vi "Loader.vi"(9 "Loader Name":string, 10 "PID":u32) -> ()   [LabVIEW 2021, in "CIFPluginLoader.lvclass"]
uses:
  CIFPluginLoader.lvclass
  CIFUtilities/CIFLogs/Typedef/Message Type.ctl
  gRPC/CIF_PluginLoader_server/RPC Messages/cif_common_Empty.ctl
  gRPC/CIF_PluginLoader_server/RPC Messages/cif_common_Status.ctl
  CIFPluginLoader.lvclass/CIFPluginLoader.ctl
  gRPC/CIF_PluginLoader_server/RPC Messages/cif_manager_LoaderStatus.ctl
  gRPC/CIF_PluginLoader_server/RPC Messages/cif_manager_LoaderInfo.ctl
  gRPC/CIF_PluginLoader_server/RPC Messages/cif_manager_LoaderType.ctl
  <vilib>/gRPC/LabVIEW gRPC Servicer/Servicer/Servicer.lvclass
  CIFUtilities/CIFLogs/CIFLogs.lvlib
  CIFUtilities/CIFConfigurationFile/typedef/Location Type.ctl
  CIFUtilities/CIFConfigurationFile/CIF Configuration File.lvlib
  <vilib>/Utility/LVLibp/NI_PackedLibraryUtility.lvlib
  gRPC/CIF_PluginLoader_server/RPC Service/PluginLoader/PluginLoader.lvclass
  gRPC/CIF_PluginLoader_server/CIF_PluginLoader_server.lvlib
  gRPC/CIF_PluginLoader_server/RPC Messages/cif_common_Version.ctl
  gRPC/CIF_PluginLoader_server/RPC Messages/cif_manager_PluginMetadata.ctl
  gRPC/CIF_PluginLoader_server/RPC Messages/cif_pluginloader_DiscoveredPlugin.ctl
  gRPC/CIF_PluginLoader_server/RPC Messages/cif_pluginloader_DiscoveredPlugins.ctl
  gRPC/CIF_Plugin_Loader_Client_Wrapper/CIFPluginLoaderClientWrapper.lvlib
panel:
  out "error out":errorcluster
  in  "stop":bool
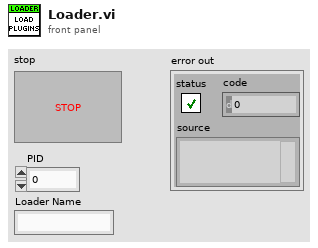
[diagram p1: front panel]
types:
  T1 = typedef "CIFLogs.lvlib/Message Type.ctl" = enum16{"Error", "Information", "Print Terminal", "Configuration"}
  T2 = typedef "CIF_PluginLoader_server.lvlib/cif_pluginloader_DiscoveredPlugins.ctl" = cluster{"discovered_plugins":T3[], "status":T6}
  T3 = typedef "CIF_PluginLoader_server.lvlib/cif_pluginloader_DiscoveredPlugin.ctl" = cluster{"file_path":string, "file_name":string, "plugin_type":string, "plugin_version":T4, "plugin_metadata":T5}
  T4 = typedef "CIF_PluginLoader_server.lvlib/cif_common_Version.ctl" = cluster{"major":u32, "minor":u32, "fix":u32, "build":u32}
  T5 = typedef "CIF_PluginLoader_server.lvlib/cif_manager_PluginMetadata.ctl" = cluster{"description":string, "history":string, "author":string}
  T6 = typedef "CIF_PluginLoader_server.lvlib/cif_common_Status.ctl" = cluster{"code":i32, "message":string}
  T7 = typedef "CIF Configuration File.lvlib/Location Type.ctl" = enum16{"Config File", "Manager", "Protos", "Plugins", "UI Plugins", "Logs", "Orchestrations"}
  T8 = typedef "CIF_PluginLoader_server.lvlib/cif_common_Empty.ctl" = cluster{"void":string}
  T9 = typedef "CIF_PluginLoader_server.lvlib/cif_manager_LoaderStatus.ctl" = cluster{"loader_info":T10, "grpc_port":i32, "pid":u32}
  T10 = typedef "CIF_PluginLoader_server.lvlib/cif_manager_LoaderInfo.ctl" = cluster{"loader_type":T11, "loader_name":string}
  T11 = typedef "CIF_PluginLoader_server.lvlib/cif_manager_LoaderType.ctl" = enum32{"LOADERTYPE_UNKNOWN", "LOADERTYPE_LABVIEW"}
  T12 = typedef "grpc-lvsupport-release.lvlib/grpcId.ctl" = u64
  T13 = typedef "CIF_PluginLoader_server.lvlib/cif_pluginloader_DiscoverCommand.ctl" = cluster{"update_metadata":bool}
  T14 = typedef "trash_Discovered Plugin.ctl" = cluster{"Filename":string, "Plugin Type":string, "Qualified name":string, "Version":T15, "Plugin Metadata":T16}
  T15 = typedef "CIFCoreCommon.lvlib/Version.ctl" = cluster{"Major":i32, "Minor":i32, "Fix":i32, "Build":i32}
  T16 = typedef "trash_Plugin Metadata.ctl" = cluster{"Description":string, "History":string, "Author":string}
  T17 = typedef "CIF_PluginLoader_server.lvlib/cif_pluginloader_LoadConfig.ctl" = cluster{"plugin_name":T18, "path":string}
  T18 = typedef "CIF_PluginLoader_server.lvlib/cif_manager_PluginName.ctl" = cluster{"plugin_name":string}
  T19 = typedef "CIFPluginLoader.lvclass/Loaded Plugin Map.ctl" = map{string, refnum<vi>}
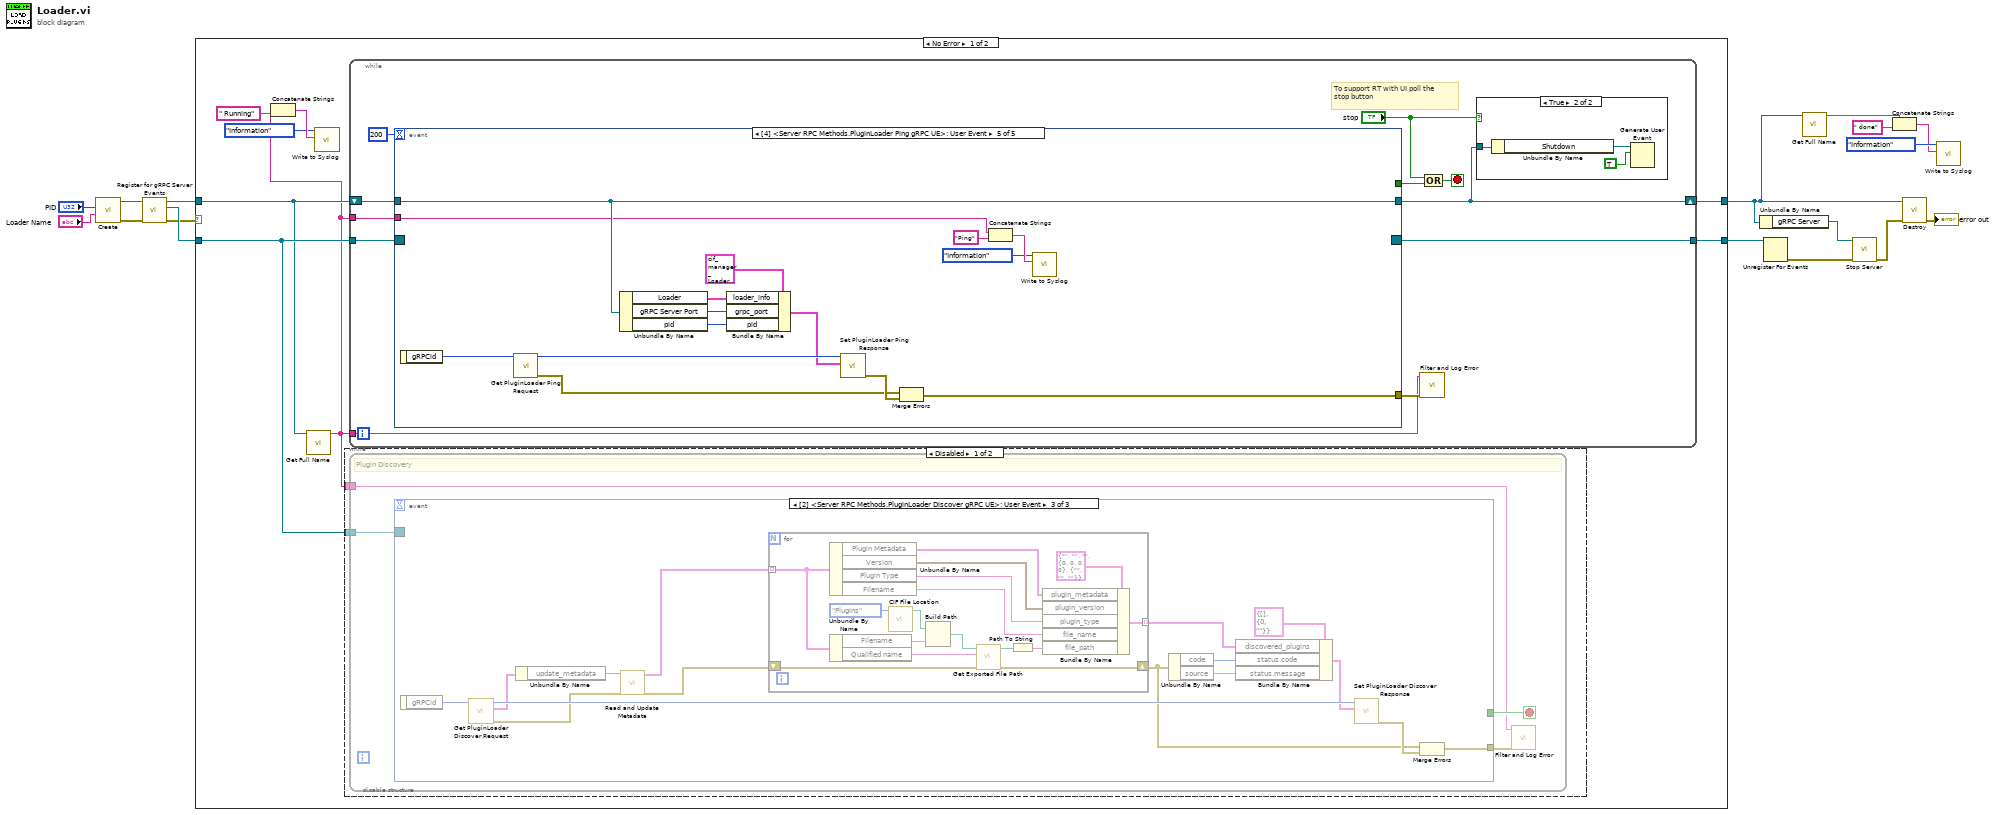
[diagram p0: block diagram]
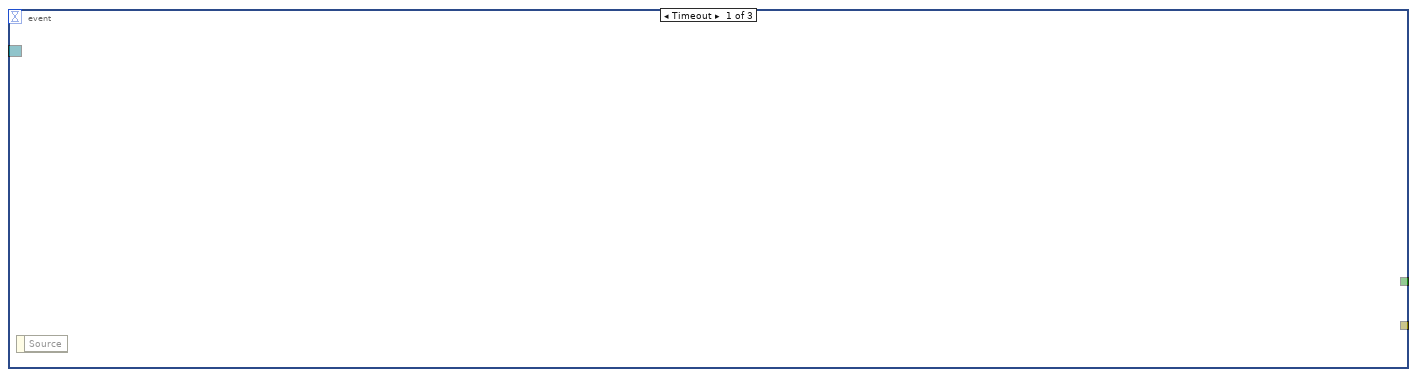
[diagram p2: hidden frame]
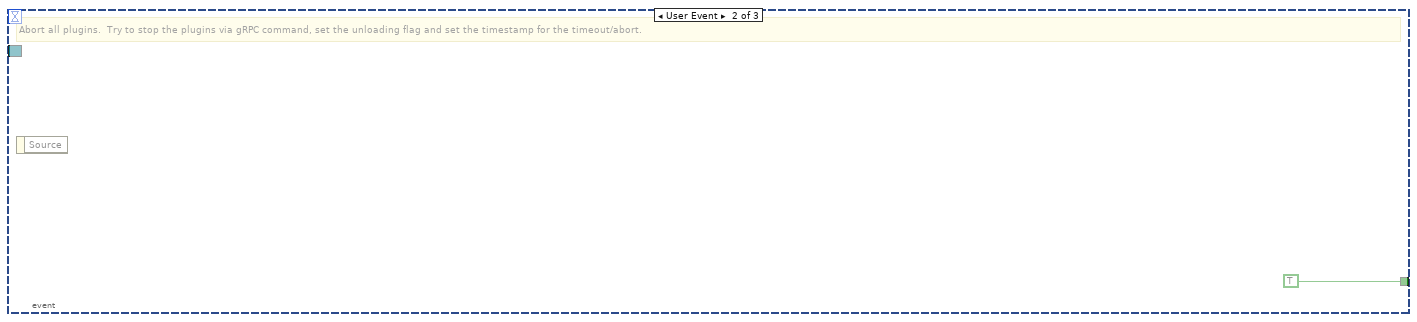
[diagram p3: hidden frame]
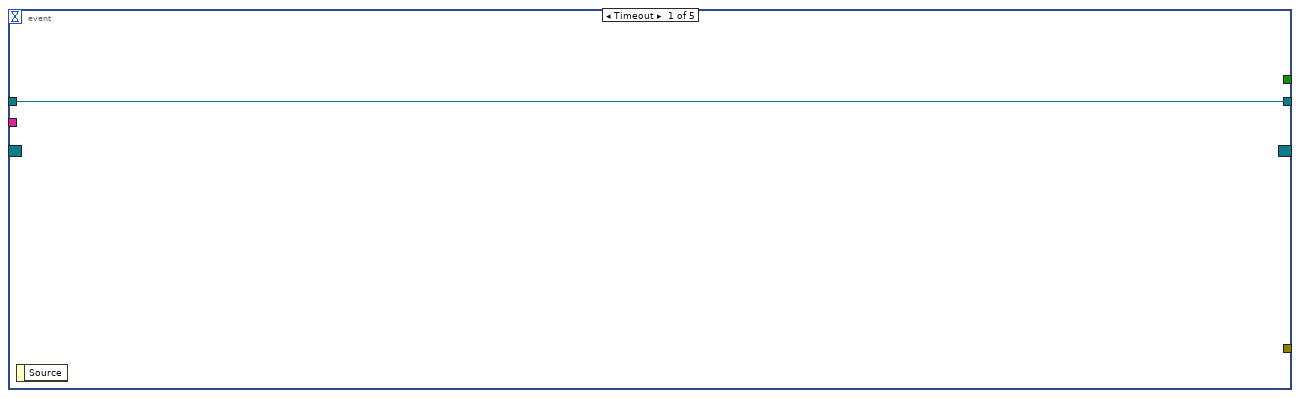
[diagram p6: hidden frame]
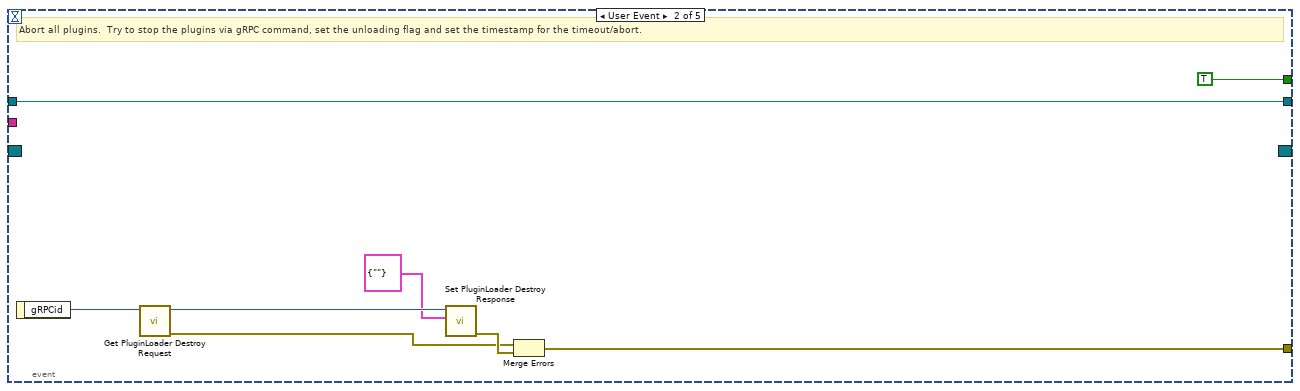
[diagram p7: hidden frame]
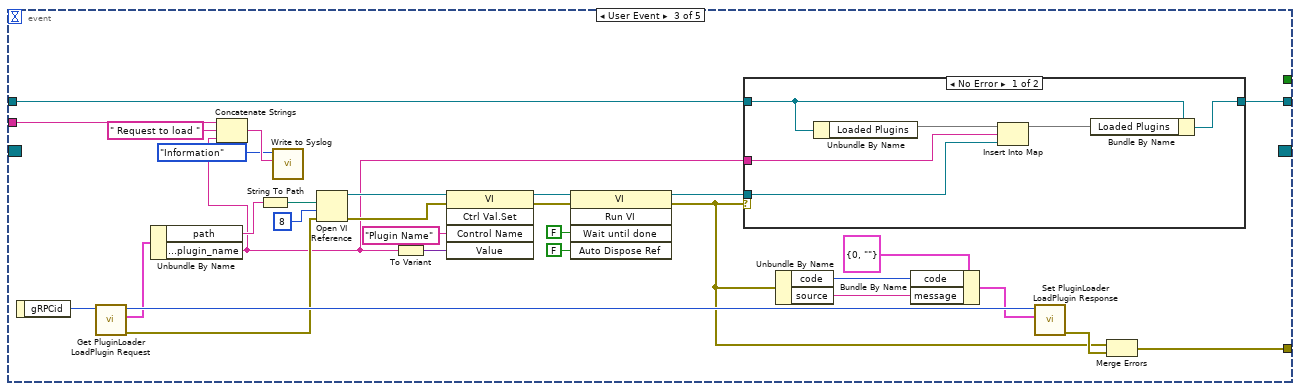
[diagram p8: hidden frame]
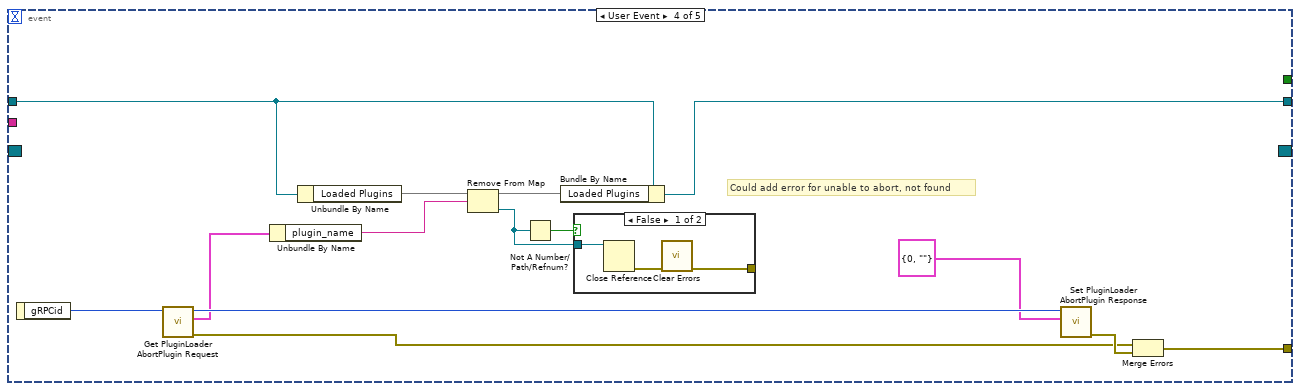
[diagram p10: hidden frame]
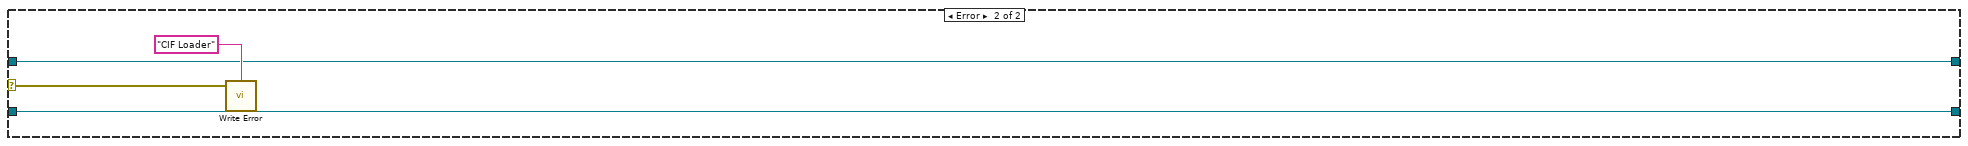
[diagram p12: hidden frame]
diagram:
  n1 = call "Create.vi"("Loader Name"="Loader Name", "pid"="PID") -> ("error out"=w12:errorcluster, "Plugin Manager out"=w8:refnum<class "CIFPluginLoader.lvclass">)  [unwired: 8 in]
  n2 = call "Register for gRPC Server Events.vi"("error in (no error)"=w12, "CIFLauncher in"=w8) -> ("error out"=w1:errorcluster, "Event Registration Refnum"=w11:refnum<event-registration>, "CIFLauncher out"=w7:refnum<class "CIFPluginLoader.lvclass">)  [unwired: 7 in]
  n3 = case shown="No Error" w1 {
    selector: w1 -> [_ w158]
    tunnel: [w25 w157] -> w2
    tunnel: [w24 w156] -> w13
    tunnel: w11 -> [w23 w156]
    tunnel: w7 -> [w22 w157]
    frame No Error {
      n4 = call "Get Full Name.vi"("CIFPluginLoader in"=w22) -> ("Full Name"=w18:string)  [unwired: 10 in]
      n5 = Concatenate Strings(w18, " Running" ("message")) -> (w21:string)
      n6 = call "Write to Syslog.vi"("message"=w21, "CIF Message Type"=Message_Type."Information") -> ()  [unwired: 9 in, 1 out]
      n7 = disable-structure shown="Disabled" {
        disable-tunnel: w23 -> [w27 _]
        disable-tunnel: w18 -> [w26 _]
        frame Disabled {
          n8 = while {
            tunnel: w27 -> [w31]
            tunnel: w26 -> [w28]
            stop <- w30 stop-if-true
            # "Plugin Discovery"
            n9 = event shown="[2] <Server RPC Methods.PluginLoader Discover gRPC UE>: User Event" {
              selector: w31 -> [_ _ _]
              dyn-events: _ -> [_ _ _]
              timeout: _ -> [_ _ _]
              tunnel: [_ _ w41] -> w29
              tunnel: [_ TRUE _] -> w30
              event Timeout {
                n10 = event-data() -> ()  [unwired: 1 in, 1 out]
              }
              event User Event {
                # "Abort all plugins.  Try to stop the plugins via gRPC command, set the unloading flag and set the timestamp for the timeout/abort."
                n11 = event-data() -> ()  [unwired: 1 in, 1 out]
              }
              event User Event {
                n12 = event-data() -> ("gRPCid"=w47:T12)  [unwired: 1 in]
                n13 = call "Get PluginLoader Discover Request.vi"("gRPCid"=w47) -> ("error out"=w43:errorcluster, "Message Data"=w45:T13, "gRPCid out"=w46:T12)  [unwired: 8 in]
                n14 = Unbundle By Name(w45) -> ("update_metadata"=w44:bool)
                n15 = call "Read and Update Metadata.vi"("error in (no error)"=w43, "Update Metadata"=w44) -> ("error out"=w39:errorcluster, "Plugin Info"=w40:T14[])  [unwired: 8 in]
                n16 = for {
                  tunnel: w40 -> [w61] mode=indexing
                  shift-right: [w62] -> w34
                  shift-left: w39 -> [w63]
                  tunnel: [w54] -> w37 mode=indexing
                  n17 = Unbundle By Name(w61) -> ("Plugin Metadata"=w55:T16, "Version"=w56:T15, "Plugin Type"=w57:string, "Filename"=w58:string)
                  n18 = Unbundle By Name(w61) -> ("Filename"=w52:string, "Qualified name"=w51:string)
                  n19 = call "CIF File Location.vi"("LocationType"=Location_Type."Plugins") -> ("Location"=w49:path)  [unwired: 10 in]
                  n20 = Build Path(base path=w49, name or relative path=w52) -> (appended path=w53:path)
                  n21 = call <vilib>:"Get Exported File Path.vi"("error in (no error)"=w63, "qualified name"=w51, "packed library path"=w53) -> ("error out"=w62:errorcluster, "path"=w60:path)  [unwired: 7 in]
                  n22 = Path To String(path=w60) -> (string=w59:string)
                  n23 = Bundle By Name(cluster=T3 {"file_path"="", "file_name"="", "plugin_type"="", "plugin_version"={"major"=0, "minor"=0, "fix"=0, "build"=0}, "plugin_metadata"={"description"="", "history"="", "author"=""}} ("cif_pluginloader_DiscoveredPlugin"), "plugin_metadata"=w55, "plugin_version"=w56, "plugin_type"=w57, "file_name"=w58, "file_path"=w59) -> (w54:T3)
                }
                n24 = Unbundle By Name(w34) -> ("code"=w38:i32, "source"=w36:string)
                n25 = Bundle By Name(cluster=T2 {"discovered_plugins"=[], "status"={"code"=0, "message"=""}} ("Message Data"), "discovered_plugins"=w37, "status.code"=w38, "status.message"=w36) -> (w35:T2)
                n26 = call "Set PluginLoader Discover Response.vi"("Message Data"=w35, "gRPCid in"=w46) -> ("error out"=w42:errorcluster)  [unwired: 9 in]
                n27 = Merge Errors(w34, w42) -> (w41:errorcluster)
              }
            }
            n28 = call "Filter and Log Error.vi"("error In"=w29, "Full Name"=w28) -> ()  [unwired: 10 in]
          }
        }
        frame Enabled {
        }
      }
      n29 = while {
        tunnel: w23 -> [w66]
        tunnel: [w73] -> w24
        shift-right: [w69] -> w25
        shift-left: w22 -> [w74]
        tunnel: w18 -> [w65]
        tunnel: w18 -> [w64]
        stop <- w71 stop-if-true
        # "To support RT with UI poll the stop button"
        n30 = event shown="[4] <Server RPC Methods.PluginLoader Ping gRPC UE>: User Event" {
          selector: w66 -> [_ _ _ _ _]
          dyn-events: [_ _ _ _ _] -> w73
          timeout: 200 -> [_ _ _ _ _]
          tunnel: w74 -> [w78 w84 w99 w130 w147]
          tunnel: [w78 w84 w97 w125 w147] -> w69
          tunnel: [_ w86 w101 w133 w152] -> w68
          tunnel: [_ TRUE _ _ _] -> w72
          tunnel: w64 -> [_ _ w88 _ w141]
          event Timeout {
            n31 = event-data() -> ()  [unwired: 1 in, 1 out]
          }
          event User Event {
            # "Abort all plugins.  Try to stop the plugins via gRPC command, set the unloading flag and set the timestamp for the timeout/abort."
            n32 = event-data() -> ("gRPCid"=w83:T12)  [unwired: 1 in]
            n33 = call "Get PluginLoader Destroy Request.vi"("gRPCid"=w83) -> ("error out"=w80:errorcluster, "gRPCid out"=w82:T12)  [unwired: 8 in, 1 out]
            n34 = call "Set PluginLoader Destroy Response.vi"("Message Data"=T8 {"void"=""}, "gRPCid in"=w82) -> ("error out"=w81:errorcluster)  [unwired: 9 in]
            n35 = Merge Errors(w80, w81) -> (w86:errorcluster)
          }
          event User Event {
            n36 = event-data() -> ("gRPCid"=w116:T12)  [unwired: 1 in]
            n37 = call "Get PluginLoader LoadPlugin Request.vi"("gRPCid"=w116) -> ("error out"=w103:errorcluster, "Message Data"=w114:T17, "gRPCid out"=w115:T12)  [unwired: 8 in]
            n38 = Unbundle By Name(w114) -> ("path"=w105:string, "plugin_name.plugin_name"=w87:string)
            n39 = Concatenate Strings(w88, " Request to load " ("message"), w87) -> (w91:string)
            n40 = String To Path(string=w105) -> (path=w104:path)
            n41 = call "Write to Syslog.vi"("message"=w91, "CIF Message Type"=Message_Type."Information") -> ()  [unwired: 9 in, 1 out]
            n42 = Open VI Reference(vi path=w104, options=8, error in (no error)=w103) -> (vi reference=w108:refnum<vi>, error out=w111:errorcluster)  [unwired: 3 in]
            n43 = To Variant(anything=w87) -> (Variant=w106:variant)
            n44 = invoke class="VI" method="Ctrl Val.Set"(reference=w108, error in=w111, "Control Name"="Plugin Name", "Value"=w106) -> (reference out=w110:refnum<vi>, error out=w109:errorcluster)  [unwired: 1 in, 3 out]
            n45 = invoke class="VI" method="Run VI"(reference=w110, error in=w109, "Wait until done"=FALSE ("Wait Until Done"), "Auto Dispose Ref"=FALSE ("Auto Dispose Reference")) -> (reference out=w98:refnum<vi>, error out=w96:errorcluster)  [unwired: 1 in, 3 out]
            n46 = case shown="No Error" w96 {
              tunnel: w99 -> [w122 w123]
              tunnel: w87 -> [w120 _]
              tunnel: w98 -> [w119 _]
              tunnel: [w117 w123] -> w97
              frame No Error {
                n47 = Unbundle By Name(w122) -> ("Loaded Plugins"=w121:T19)
                n48 = Insert Into Map(map in=w121, key=w120, value=w119) -> (map out=w118:T19)  [unwired: 2 out]
                n49 = Bundle By Name(cluster=w122, "Loaded Plugins"=w118) -> (w117:refnum<class "CIFPluginLoader.lvclass">)
              }
              frame Error {
              }
            }
            n50 = Unbundle By Name(w96) -> ("code"=w94:i32, "source"=w95:string)
            n51 = Bundle By Name(cluster=T6 {"code"=0, "message"=""} ("Message Data"), "code"=w94, "message"=w95) -> (w93:T6)
            n52 = call "Set PluginLoader LoadPlugin Response.vi"("Message Data"=w93, "gRPCid in"=w115) -> ("error out"=w102:errorcluster)  [unwired: 9 in]
            n53 = Merge Errors(w96, w102) -> (w101:errorcluster)
          }
          event User Event {
            # "Could add error for unable to abort, not found"
            n54 = event-data() -> ("gRPCid"=w137:T12)  [unwired: 1 in]
            n55 = call "Get PluginLoader AbortPlugin Request.vi"("gRPCid"=w137) -> ("error out"=w132:errorcluster, "Message Data"=w135:T18, "gRPCid out"=w136:T12)  [unwired: 8 in]
            n56 = Unbundle By Name(w135) -> ("plugin_name"=w127:string)
            n57 = Unbundle By Name(w130) -> ("Loaded Plugins"=w128:T19)
            n58 = Remove From Map(10:w127, 11:w128) -> (1:w126:refnum<vi>, 3:w129:T19)  [unwired: 1 out]
            n59 = Not A Number/Path/Refnum?(number/path/refnum=w126) -> (NaN/Path/Refnum?=w131:bool)
            n60 = Bundle By Name(cluster=w130, "Loaded Plugins"=w129) -> (w125:refnum<class "CIFPluginLoader.lvclass">)
            n61 = case shown="False" w131 {
              tunnel: w126 -> [w140 _]
              tunnel: [w138 _] -> _
              frame False {
                n62 = Close Reference(reference=w140) -> (error out=w139:errorcluster)  [unwired: 1 in]
                n63 = call <vilib>:"Clear Errors.vi"("error in (no error)"=w139) -> ("error out"=w138:errorcluster)  [unwired: 5 in, 1 out]
              }
              frame True {
              }
            }
            n64 = call "Set PluginLoader AbortPlugin Response.vi"("Message Data"=T6 {"code"=0, "message"=""}, "gRPCid in"=w136) -> ("error out"=w134:errorcluster)  [unwired: 9 in]
            n65 = Merge Errors(w132, w134) -> (w133:errorcluster)
          }
          event User Event {
            n66 = event-data() -> ("gRPCid"=w155:T12)  [unwired: 1 in]
            n67 = call "Get PluginLoader Ping Request.vi"("gRPCid"=w155) -> ("error out"=w151:errorcluster, "gRPCid out"=w154:T12)  [unwired: 8 in, 1 out]
            n68 = Unbundle By Name(w147) -> ("Loader"=w150:T10, "gRPC Server Port"=w149:i32, "pid"=w148:u32)
            n69 = Bundle By Name(cluster=T9 {"loader_info"={"loader_type"=enum."LOADERTYPE_UNKNOWN", "loader_name"=""}, "grpc_port"=0, "pid"=0} ("Message Data"), "loader_info"=w150, "grpc_port"=w149, "pid"=w148) -> (w145:T9)
            n70 = call "Set PluginLoader Ping Response.vi"("Message Data"=w145, "gRPCid in"=w154) -> ("error out"=w153:errorcluster)  [unwired: 9 in]
            n71 = Merge Errors(w151, w153) -> (w152:errorcluster)
            n72 = Concatenate Strings(w141, "Ping" ("message")) -> (w144:string)
            n73 = call "Write to Syslog.vi"("message"=w144, "CIF Message Type"=Message_Type."Information") -> ()  [unwired: 9 in, 1 out]
          }
        }
        n74 = call "Filter and Log Error.vi"("error In"=w68, "Full Name"=w65) -> ()  [unwired: 10 in]
        n75 = Compound Arithmetic op=OR("stop", w72) -> (w71:bool)
        n76 = case shown="True" "stop" {
          tunnel: w69 -> [_ w75]
          frame False {
          }
          frame True {
            n77 = Unbundle By Name(w75) -> ("Shutdown"=w76:refnum<user-event>)
            n78 = Generate User Event(user event=w76, event data cluster=TRUE ("event data")) -> ()  [unwired: 2 in, 2 out]
          }
        }
      }
    }
    frame Error {
      n79 = call "Write Error.vi"("error in (no error)"=w158, "Plugin Name"="CIF Loader") -> ()  [unwired: 2 in, 1 out]
    }
  }
  n80 = Unbundle By Name(w2) -> ("gRPC Server"=w16:refnum<class "Servicer.lvclass">)
  n81 = Unregister For Events(event registration refnum=w13) -> (error out=w17:errorcluster)  [unwired: 1 in]
  n82 = call "Get Full Name.vi"("CIFPluginLoader in"=w2) -> ("Full Name"=w3:string)  [unwired: 10 in]
  n83 = call <vilib>:"Stop Server.vi"("error in"=w17, "gRPC Server in"=w16) -> ("error out"=w15:errorcluster)  [unwired: 9 in]
  n84 = Concatenate Strings(w3, " done" ("message")) -> (w4:string)
  n85 = call "Destroy.vi"("error in (no error)"=w15, "Plugin Manager in"=w2) -> ("error out"=→"error out":errorcluster)  [unwired: 8 in, 1 out]
  n86 = call "Write to Syslog.vi"("message"=w4, "CIF Message Type"=Message_Type."Information") -> ()  [unwired: 9 in, 1 out]
